vi "GetBounds.vi"(0 "XRef":T14, 1 "State In":T4) -> (14 "Bounds":T2, 15 "Fatal Error Out":T1)   [LabVIEW 2020, in "Parallel Diagram Block.xnode"]
uses:
  Parallel Diagram Block.xnode
  <vilib>/XNodeSupport/XNodeXNodeRef.ctl
  State.ctl
  Parallel Block/Type Descriptor.ctl
  Parallel Block/Direction.ctl
  Parallel Block/Value Type.ctl
  Parallel Block/Terminal Mode.ctl
  Parallel Block/Terminal Type.ctl
  <vilib>/picture/picture.llb/imagedata.ctl
  <vilib>/XNodeSupport/XNodeBounds.ctl
  <vilib>/XNodeSupport/XNodeInt.ctl
  <vilib>/XNodeSupport/XNodeErrorCluster.ctl
  <vilib>/XNodeSupport/NI_XNodeSupport.lvlib
  Parallel Block/Parallel Block.lvlib
  Parallel Block/Type Mode.ctl
  Parallel Block/Value Mode.ctl
  Parallel Block/Manager Node.ctl
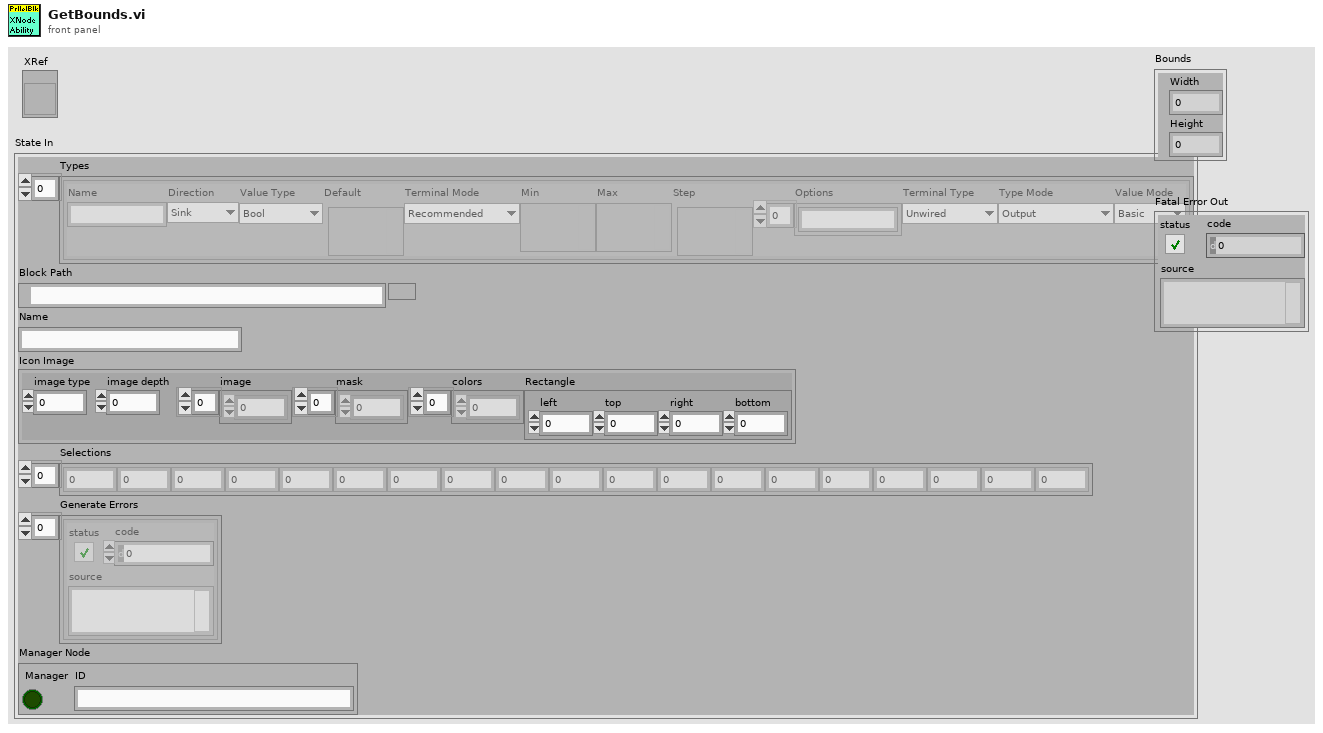
[diagram p1: front panel]
types:
  T1 = typedef "NI_XNodeSupport.lvlib/XNodeErrorCluster.ctl" = errorcluster
  T2 = typedef "NI_XNodeSupport.lvlib/XNodeBounds.ctl" = cluster{"Width":T3, "Height":T3}
  T3 = typedef "NI_XNodeSupport.lvlib/XNodeInt.ctl" = i32
  T4 = typedef "Parallel Diagram Block.xnode/State.ctl" = cluster{"Types":T5[], "Block Path":path, "Name":string, "Icon Image":T12, "Selections":i32[], "Generate Errors":errorcluster[], "Manager Node":T13}
  T5 = typedef "Parallel Block.lvlib/Type Descriptor.ctl" = cluster{"Name":string, "Direction":T6, "Value Type":T7, "Default":variant, "Terminal Mode":T8, "Min":variant, "Max":variant, "Step":variant, "Options":string[], "Terminal Type":T9, "Type Mode":T10, "Value Mode":T11}
  T6 = typedef "Parallel Block.lvlib/Direction.ctl" = enum16{"Sink", "Source"}
  T7 = typedef "Parallel Block.lvlib/Value Type.ctl" = enum16{"Unknown", "Bool", "U8", "U16", "U32", "U64", "I8", "I16", "I32", "I64", "SGL", "DBL", "CSG", "CDB", "CDBWfm", "String", "DBLWfm"}
  T8 = typedef "Parallel Block.lvlib/Terminal Mode.ctl" = enum16{"Recommended", "Required", "None"}
  T9 = typedef "Parallel Block.lvlib/Terminal Type.ctl" = enum16{"Unwired", "BadType", "Connection", "Value", "Control Ref", "BadRefType"}
  T10 = typedef "Parallel Block.lvlib/Type Mode.ctl" = enum16{"Output", "Single - Strict", "Single - Coerced", "Stream"}
  T11 = typedef "Parallel Block.lvlib/Value Mode.ctl" = enum16{"Basic", "Range", "Select"}
  T12 = typedef "imagedata.ctl" = cluster{"image type":i32, "image depth":i32, "image":u8[], "mask":u8[], "colors":u32[], "Rectangle":cluster{"left":i16, "top":i16, "right":i16, "bottom":i16}}
  T13 = typedef "Parallel Block.lvlib/Manager Node.ctl" = cluster{"Manager":bool, "ID":string}
  T14 = typedef "NI_XNodeSupport.lvlib/XNodeXNodeRef.ctl" = refnum<vi>
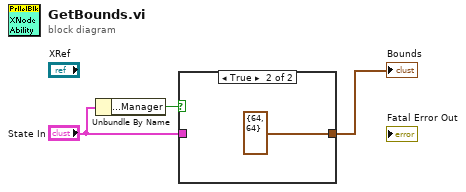
[diagram p0: block diagram]
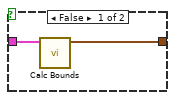
[diagram p2: hidden frame]
diagram:
  n1 = Unbundle By Name("State In") -> ("Manager Node.Manager"=w1:bool)
  n2 = case shown="True" w1 {
    tunnel: [w5 T2 {"Width"=64, "Height"=64} ("Text Bounds")] -> w3
    tunnel: "State In" -> [w4 _]
    frame False {
      n3 = call "Calc Bounds.vi"("State"=w4) -> ("Text Bounds"=w5:T2)  [unwired: 4 in, 6 out]
    }
    frame True {
    }
  }
  "Bounds" <- w3
